vi "[NameData] - Strings from Variants.vi"(4 "Format Cluster":T2, 6 "String Format Select":T1, 7 "Section Name (Name Of \"Anything\")":string, 8 "Error":errorcluster, 9 "Remove Source Name":bool, 11 "Anything":variant) -> (0 "Error Out":errorcluster, 1 "Name Val 2d Array Out":string[][](array[string]), 2 "Values Out":string[](array[string]), 3 "Names Out":string[](array[string]), 5 "Section Out":string)   [LabVIEW 2020]
uses:
  TypeDefs_Utility/Cluster_NameData_String Format Data.ctl
  TypeDefs_Utility/ENUM_NameData_String Format Select.ctl
  <vilib>/Utility/Data Type/NI_Data Type.lvlib
panel:
  # "%.2f %g %e %p"
  # "%d %h %o %b"
  # "'%s'"
  # "%x %X"
  # "True,False -1,0 Yes,No"
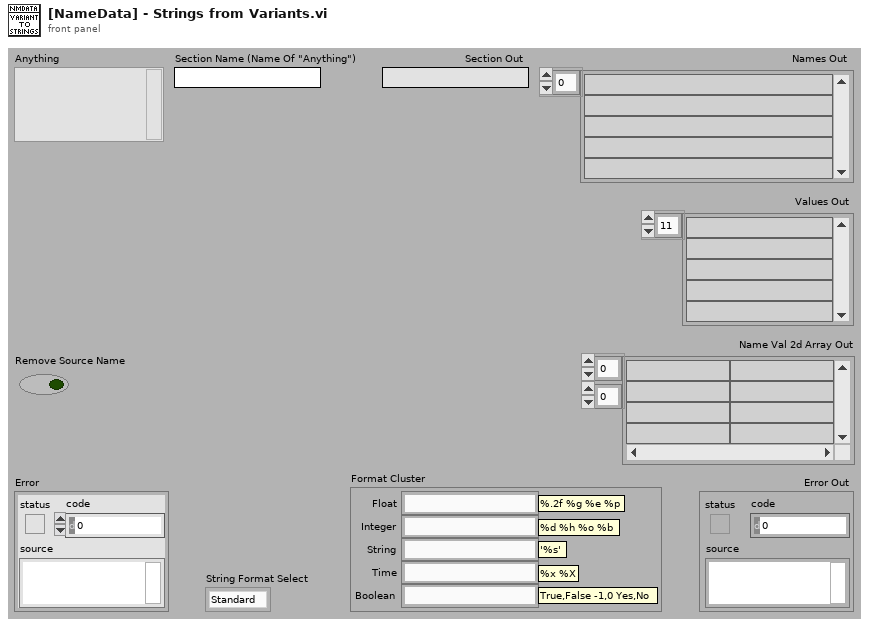
[diagram p1: front panel]
types:
  T1 = typedef "ENUM_NameData_String Format Select.ctl" = enum16{"Standard", "Access DB", "Custom"}
  T2 = typedef "Cluster_NameData_String Format Data.ctl" = cluster{"Float":string, "Integer":string, "String":string, "Time":string, "Boolean":string}
  T3 = typedef "NI_Data Type.lvlib/Data Type.ctl" = enum8{"Invalid Type", "Void", "I8", "I16", "I32", "I64", "U8", "U16", "U32", "U64", "Single Float", "Double Float", "Extended Float", "Single Complex", "Double Complex", "Extended Complex", "Enum U8", "Enum U16", "Enum U32", "Enum U64", "Single Float With Unit", "Double Float With Unit", "Extended Float With Unit", "Single Complex with Unit", "Double Complex with Unit", "Extended Complex with Unit", "Boolean", "String", "Path", "Picture", "Tag", "Array", "Cluster", "Variant", "LV Variant", "Waveform", "Timestamp", "Digital Waveform", "Digital Data", "ExpressData", "Refnum", "External Data", "VI", "Poly VI", "LabVIEW Class Instance", "Fixed Point", "Set Collection", "Map Collection"}
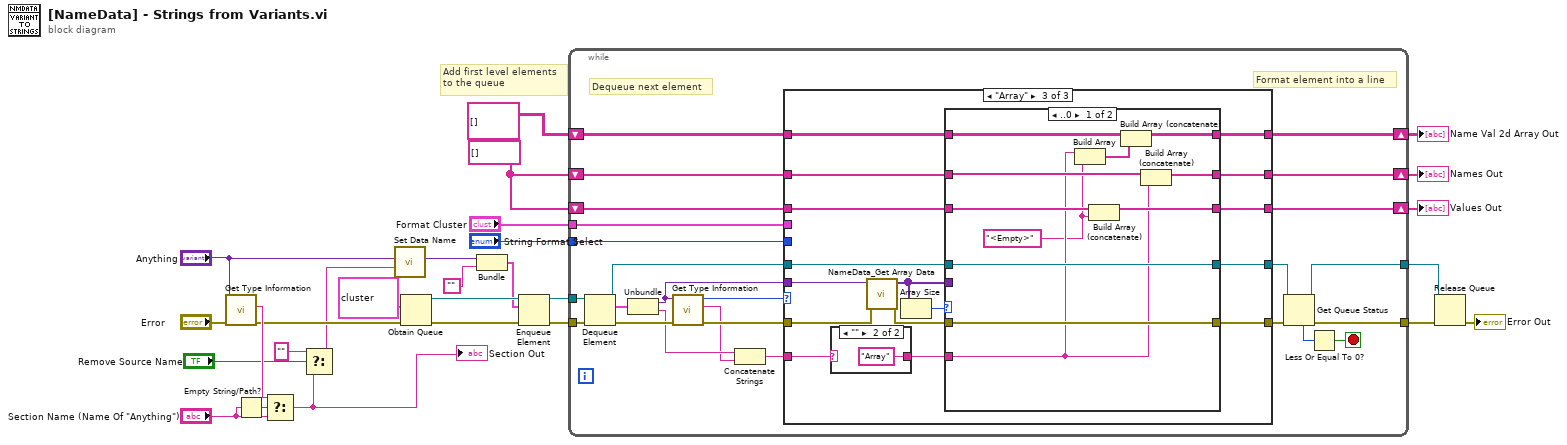
[diagram p0: block diagram]
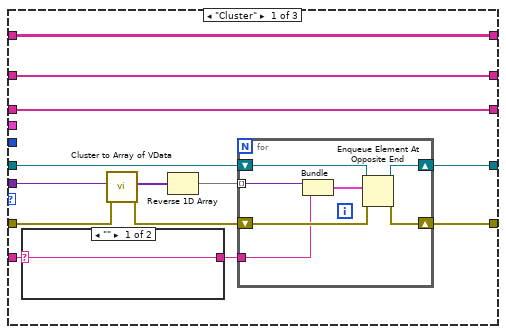
[diagram p2: hidden frame]
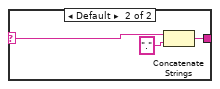
[diagram p3: hidden frame]
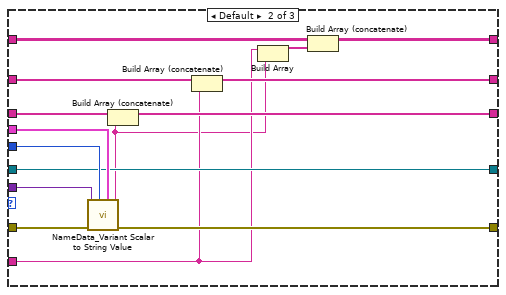
[diagram p4: hidden frame]
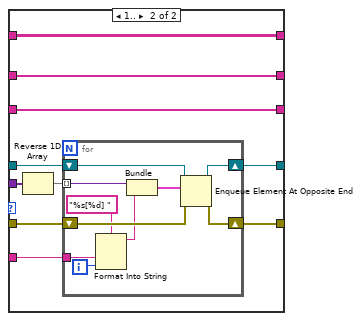
[diagram p6: hidden frame]
diagram:
  w15 = string[] []
  # "Add first level elements\nto the queue"
  n1 = call <vilib>:"Get Type Information.vi"("error in (no error)"="Error", "variant"="Anything") -> ("error out"=w10:errorcluster, "name"=w19:string)  [unwired: 5 in, 3 out]
  n2 = Empty String/Path?(string/path="Section Name (Name Of \"Anything\")") -> (empty?=w20:bool)
  n3 = Select(t=w19, s=w20, f="Section Name (Name Of \"Anything\")") -> (s? t:f=w4:string)
  "Section Out" <- w4
  n4 = Select(t="", s="Remove Source Name", f=w4) -> (s? t:f=w5:string)
  n5 = call "Set Data Name.vi"("Data Name"=w5, "Data"="Anything") -> ("Renamed Data"=w7:variant)  [unwired: 8 in, 1 out]
  n6 = Obtain Queue(element data type=cluster{"Variant":variant, "Name":string} {"Variant"=variant, "Name"=""}, error in (no error)=w10) -> (queue out=w28:refnum<queue>, error out=w27:errorcluster)  [unwired: 3 in, 1 out]
  n7 = Bundle("Renamed Data"=w7, "") -> (w17:cluster{"Renamed Data":variant, string})  [unwired: 1 in]
  n8 = Enqueue Element(queue=w28, element=w17, error in (no error)=w27) -> (queue out=w25:refnum<queue>, error out=w26:errorcluster)  [unwired: 1 in, 1 out]
  n9 = while {
    tunnel: w26 -> [w53]
    tunnel: [w50] -> w24
    tunnel: w25 -> [w51]
    tunnel: [w47] -> w23
    shift-right: [w39] -> w11
    shift-left: w15 -> [w34]
    shift-right: [w38] -> w12
    shift-left: w15 -> [w35]
    tunnel: "Format Cluster" -> [w33]
    tunnel: "String Format Select" -> [w32]
    shift-right: [w29] -> w1
    shift-left: string[][] [] -> [w30]
    stop <- w48 stop-if-true
    # "Format element into a line"
    # "Dequeue next element"
    n10 = Dequeue Element(queue=w51, error in (no error)=w53) -> (queue out=w45:refnum<queue>, element=w43:cluster{"Variant":variant, "Name":string}, error out=w52:errorcluster)  [unwired: 1 in, 1 out]
    n11 = Unbundle(w43) -> ("Variant"=w42:variant, "Name"=w41:string)
    n12 = call <vilib>:"Get Type Information.vi"("error in (no error)"=w52, "variant"=w42) -> ("error out"=w40:errorcluster, "name"=w31:string, "type"=w36:T3)  [unwired: 5 in, 2 out]
    n13 = Concatenate Strings(w41, w31) -> (w37:string)
    n14 = case shown="\"Array\"" w36 {
      tunnel: [w66 w83 w105] -> w46
      tunnel: w45 -> [w65 w83 w106]
      tunnel: [w64 w92 w103] -> w44
      tunnel: w42 -> [w63 w86 w107]
      tunnel: w40 -> [w62 w87 w108]
      tunnel: [w56 w89 w99] -> w39
      tunnel: [w57 w90 w98] -> w38
      tunnel: w37 -> [w55 w82 w96]
      tunnel: w35 -> [w57 w91 w101]
      tunnel: w34 -> [w56 w88 w100]
      tunnel: w33 -> [_ w84 _]
      tunnel: w32 -> [_ w85 _]
      tunnel: w30 -> [w54 w79 w94]
      tunnel: [w54 w78 w93] -> w29
      frame "Cluster" {
        n15 = case shown="\"\"" w55 {
          selector: w55 -> [w67 w68]
          tunnel: [w67 w69] -> w58
          frame "" {
          }
          frame Default {
            n16 = Concatenate Strings(w68, "." ("string")) -> (w69:string)
          }
        }
        n17 = call "Cluster to Array of VData.vi"("error in (no error)"=w62, "Cluster"=w63) -> ("error out"=w60:errorcluster, "Array of VData"=w59:variant[])  [unwired: 8 in]
        n18 = Reverse 1D Array(array=w59) -> (reversed array=w61:variant[])
        n19 = for {
          tunnel: w61 -> [w72] mode=indexing
          tunnel: w58 -> [w71]
          shift-right: [w74] -> w66
          shift-left: w65 -> [w77]
          shift-right: [w75] -> w64
          shift-left: w60 -> [w76]
          n20 = Bundle("Variant"=w72, w71) -> (w73:cluster{"Variant":variant, string})  [unwired: 1 in]
          n21 = Enqueue Element At Opposite End(queue=w77, element=w73, error in (no error)=w76) -> (queue out=w74:refnum<queue>, error out=w75:errorcluster)  [unwired: 1 in, 1 out]
        }
      }
      frame Default {
        n22 = call "NameData_Variant Scalar to String Value.vi"("Format Cluster"=w84, "String Format Select"=w85, "Error"=w87, "Variant"=w86) -> ("Error Out"=w92:errorcluster, "Value Out"=w81:string)  [unwired: 5 in, 1 out]
        n23 = Build Array (concatenate)(w88, w81) -> (w89:string[])
        n24 = Build Array (concatenate)(w91, w82) -> (w90:string[])
        n25 = Build Array(w82, w81) -> (w80:string[])
        n26 = Build Array (concatenate)(w79, w80) -> (w78:string[][])
      }
      frame "Array" {
        n27 = case shown="\"\"" w96 {
          selector: w96 -> [w109 _]
          tunnel: [w109 "Array"] -> w95
          frame Default {
          }
          frame "" {
          }
        }
        n28 = call "NameData_Get Array Data.vi"("Error"=w108, "Array Variant"=w107) -> ("Error Out"=w104:errorcluster, "Data Array Out"=w102:variant[])  [unwired: 7 in, 1 out]
        n29 = Array Size(array=w102) -> (size(s)=w97:i32)
        n30 = case shown="..0" w97 {
          tunnel: w106 -> [w117 w131]
          tunnel: [w117 w130] -> w105
          tunnel: w95 -> [w115 w129]
          tunnel: w104 -> [w116 w128]
          tunnel: [w116 w127] -> w103
          tunnel: w102 -> [_ w125]
          tunnel: w101 -> [w121 w123]
          tunnel: w100 -> [w119 w124]
          tunnel: [w118 w124] -> w99
          tunnel: [w120 w123] -> w98
          tunnel: w94 -> [w112 w122]
          tunnel: [w111 w122] -> w93
          frame ..0 {
            w114 = "<Empty>"
            n31 = Build Array(w115, w114) -> (w113:string[])
            n32 = Build Array (concatenate)(w119, w114) -> (w118:string[])
            n33 = Build Array (concatenate)(w112, w113) -> (w111:string[][])
            n34 = Build Array (concatenate)(w121, w115) -> (w120:string[])
          }
          frame 1.. {
            n35 = Reverse 1D Array(array=w125) -> (reversed array=w126:variant[])
            n36 = for {
              tunnel: w126 -> [w136] mode=indexing
              tunnel: w129 -> [w134]
              shift-right: [w138] -> w130
              shift-left: w131 -> [w141]
              shift-right: [w139] -> w127
              shift-left: w128 -> [w140]
              i -> [w133]
              n37 = Format Into String(format string="%s[%d] ", w134, w133) -> (resulting string=w132:string)  [unwired: 2 in, 1 out]
              n38 = Bundle("Variant"=w136, w132) -> (w137:cluster{"Variant":variant, string})  [unwired: 1 in]
              n39 = Enqueue Element At Opposite End(queue=w141, element=w137, error in (no error)=w140) -> (queue out=w138:refnum<queue>, error out=w139:errorcluster)  [unwired: 1 in, 1 out]
            }
          }
        }
      }
    }
    n40 = Get Queue Status(queue=w46, error in (no error)=w44) -> (queue out=w47:refnum<queue>, error out=w50:errorcluster, # elements in queue=w49:i32)  [unwired: 1 in, 5 out]
    n41 = Less Or Equal To 0?(x=w49) -> (x <= 0?=w48:bool)
  }
  "Names Out" <- w12
  "Values Out" <- w11
  "Name Val 2d Array Out" <- w1
  n42 = Release Queue(queue=w23, error in (no error)=w24) -> (error out=→"Error Out":errorcluster)  [unwired: 1 in, 2 out]
